vi "GLOBAL_heating_indicator.vi"() -> ()   [LabVIEW 2021]
panel:
  out "TRAP IS HEATING":bool
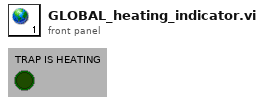
[diagram p1: front panel]
diagram:
